vi "algo1.vi"() -> ()   [LabVIEW 2015]
uses:
  <vilib>/vision/Image Controls.llb/IMAQ Image.ctl
panel:
  out "New Image":T1
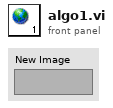
[diagram p1: front panel]
types:
  T1 = typedef "IMAQ Image.ctl" = refnum<image>
diagram:
